vi "Laurel Rate Total TCP.vi"(6 "Laurel Communication Type":string, 8 "error in (no error)":errorcluster, 10 "Measurments in":T7={"Power Measurements"={"Current (A):Element 1"=0.0, "Current (A):Element 2"=0.0, "Power (W):Sigma"=0.0, "Watt Hours (Wh):Sigma"=0.0, "Voltage (V):Element 2"=0.0, "Voltage (V):Element 1"=0.0, "Current Crest Factor:Element 1"=0.0, "Current Crest Factor:Element 2"=0.0, "Voltage Harmonic (%):Element 1"=0.0, "Voltage Harmonic (%):Element 2"=0.0, "Voltage Crest Factor:Element 1"=0.0, "Voltage Crest Factor:Element 2"=0.0, "Time:Element 1"=0.0, "Frequency (Hz):Element 1"=0.0, "Apparent Power (VA):Element 1"=0.0, "Apparent Power (VA):Element 2"=0.0, "Power Factor:Element 1"=0.0, "Power Factor:Element 2"=0.0, "Max Watt Hours"=0.0, "Voltage (V):Element 2 Avg"=0.0, "Voltage (V):Element 1 Avg"=0.0}, "Standby Power"={"Standby Power Spreadsheet"=[], "Standby Power - Pia (Watts)"=0.0, "Off Mode Power - Poff (Watts)"=0.0, "Sia hr/yr"=8620.0, "Soff hr/yr"=0.0, "Yearly Energy Etso kWh/yr"=0.0, "Maximum Power (Watts)"=0.0, "Power Variation (%)"=0.0, "Slope (mW/hr)"=0.0, "Final Harmonics-U1 (%)"="", "Final Harmonics-U2 (%)"="", "Energy (Wh)"=0.0}, "Washer"={"Washer String Data"=[], "Analog Scale Weight (lbs)"=0.0}, "Dishwasher"={"Drain Solonoid Event"=0, "Pump Event"=0, "Water Valve Event"=0, "Heater Event"=0, "Motor Event"=0, "Turbidity Sensor"=0.0, "Spare 2"=0.0, "Spare 3"=0.0, "Spare 4"=0.0, "Spare 5"=0.0, "Thermocouple 1"=0.0, "Thermocouple 2"=0.0, "Thermocouple 3"=0.0, "Thermocouple 4"=0.0, "Thermocouple 5"=0.0, "Thermocouple 6"=0.0, "Spare 1"=0.0, "Dishwasher String Data"=[]}, "Washer HCC"={"Chan 101"=0.0, "Chan 102"=0.0, "Chan 103"=0.0, "Chan 104"=0.0, "Chan 105"=0.0, "Chan 106"=0.0, "Chan 107"=0.0, "Chan 108"=0.0, "Chan 109"=0.0, "Chan 110"=0.0, "Chan 111"=0.0, "Chan 112"=0.0, "Chan 113"=0.0, "Chan 114"=0.0, "Chan 115"=0.0, "Chan 116"=0.0, "Chan 117"=0.0, "Chan 118"=0.0, "Chan 119"=0.0, "Chan 120"=0.0, "Chan 201"=0.0, "Chan 202"=0.0, "Chan 203"=0.0, "Chan 204"=0.0, "Chan 205"=0.0, "Chan 206"=0.0, "Chan 207"=0.0, "Chan 208"=0.0, "Chan 209"=0.0, "Chan 210"=0.0, "Chan 211"=0.0, "Chan 212"=0.0, "Chan 213"=0.0, "Chan 214"=0.0, "Chan 215"=0.0, "Chan 216"=0.0, "Chan 217"=0.0, "Chan 218"=0.0, "Chan 219"=0.0, "Chan 220"=0.0, "Chan 301"=0.0, "Chan 302"=0.0, "Chan 303"=0.0, "Chan 304"=0.0, "Chan 305"=0.0, "Chan 306"=0.0, "Chan 307"=0.0, "Chan 308"=0.0, "Chan 309"=0.0, "Chan 310"=0.0, "Chan 311"=0.0, "Chan 312"=0.0, "Chan 313"=0.0, "Chan 314"=0.0, "Chan 315"=0.0, "Chan 316"=0.0, "Chan 317"=0.0, "Chan 318"=0.0, "Chan 319"=0.0, "Chan 320"=0.0}, "Barometric Pressure"={"Barometric Pressure (in. Hg)"=0.0}, "Ambient Conditions"={"Ambient Temperature  1 (°F)"=0.0, "Ambient Temperature 2 (°F)"=0.0, "Ambient Temperature 3 (°F)"=0.0, "Ambient Humidity 1 (%)"=0.0, "Ambient Humidity 2 (%)"=0.0, "Ambient Humidity 3 (%)"=0.0, "Ambient Dewpoint  1 (°F)"=0.0, "Ambient Dewpoint 2 (°F)"=0.0, "Ambient Dewpoint 3 (°F)"=0.0}, "Weight Scale"={"Gross Weigth (lbs)"=0.0, "Net Weight (lbs)"=0.0, "Final Weight (lbs)"=""}, "Water Measurements"={"Hot Water Pressure (psi)"=0.0, "Hot Water Pressure Max (psi)"=0.0, "Hot Water Temperature (°F)"=0.0, "Cold Water Pressure (psi)"=0.0, "Cold Water Pressure Max (psi)"=0.0, "Hot Water Temperature Max (°F)"=0.0, "Cold Water Temperature (°F)"=0.0, "Cold Water Temperature Max (°F)"=0.0, "Hot Water Total (Gal)"=0.0, "Hot Water Rate (GPM)"=0.0, "Cold Water Total (Gal)"=0.0, "Cold Water Rate (GPM)"=0.0, "Cold Water Total During Wash (Gal)"=0.0, "Hot Water Total During Wash (Gal)"=0.0, "Rinse Cold (Gal)"=0.0, "Rinse Hot (Gal)"=0.0, "Hot Water Pressure Min (psi)"=0.0, "Hot Water Temperature Min (°F)"=0.0, "Cold Water Pressure Min (psi)"=0.0, "Cold Water Temperature Min (°F)"=0.0}, "Gas Data"={"Meter Type (Gas)"="", "Meter ID"=enum."Disabled", "Heating Value (BTU/ft³)"=0.0, "Ft³ / Hr (SCFH)"=0.0, "15 Second Average (BTU/HR)"=0.0, "30 Second Average (BTU/HR)"=0.0, "SLPM (Mass Flow)"=0.0, "LPM (Vol. Flow)"=0.0, "Gas Temperature (°F)"=0.0, "Gas Pressure (PSIA)"=0.0, "Tot.Flow (Liters)"=0.0}} {"Power Measurements"."Voltage (V):Element 1 Avg" format="%.3g"; "Power Measurements"."Voltage (V):Element 2 Avg" format="%.3g"; "Power Measurements"."Max Watt Hours" format="%.3g"; "Power Measurements"."Power Factor:Element 2" format="%.3g"; "Power Measurements"."Power Factor:Element 1" format="%.3g"; "Power Measurements"."Apparent Power (VA):Element 2" format="%.3g"; "Power Measurements"."Apparent Power (VA):Element 1" format="%.3g"; "Power Measurements"."Frequency (Hz):Element 1" format="%.3g"; "Power Measurements"."Time:Element 1" format="%.3g"; "Power Measurements"."Voltage Crest Factor:Element 2" format="%.3g"; "Power Measurements"."Voltage Crest Factor:Element 1" format="%.3g"; "Power Measurements"."Voltage Harmonic (%):Element 2" format="%.3g"; "Power Measurements"."Voltage Harmonic (%):Element 1" format="%.3g"; "Power Measurements"."Current Crest Factor:Element 2" format="%.3g"; "Power Measurements"."Current Crest Factor:Element 1" format="%.3g"; "Power Measurements"."Voltage (V):Element 1" format="%.3g"; "Power Measurements"."Voltage (V):Element 2" format="%.3g"; "Power Measurements"."Watt Hours (Wh):Sigma" format="%.3f"; "Power Measurements"."Power (W):Sigma" format="%.3g"; "Power Measurements"."Current (A):Element 2" format="%.3g"; "Power Measurements"."Current (A):Element 1" format="%.3g"}, 11 "Fixture Hardware in":T1={"Power "={"Yokogawa"={"WT210"={"Sample Rate (1: 0.25s)"=0, "A Range (12: 20A)"=0, "V Range (6: 600V)"=0, "Power VISA Yokogawa WT210"=""}, "WT500"={"Power VISA Yokogawa WT500"="", "V Range (8: 1000V)"=0, "I Range (7: 40A)"=0, "Update Rate (3: 500ms)"=0}, "WT310_2"={"Sample Rate (1: 0.25s)"=1, "A Range (12: 20A)"=11, "V Range (6: 600V)"=4, "Power VISA Yokogawa WT310_2"=""}, "WT310_3"={"Sample Rate (1: 0.25s)"=1, "A Range (12: 20A)"=11, "V Range (6: 600V)"=4, "Power VISA Yokogawa WT310_3"=""}}, "Aplus"={"Aplus IP Address"="", "Remote Port"=0, "Instrument"="", "Instr Driver Revision"=""}, "Power Limits"={"Crest Factor"={"Upper Limit"=0.0, "Lower Limit"=0.0}, "Harmonic Content"={"Uthd"=0.0}, "Voltage"={"% Error"=0.0}, "Stability"={"<1 Watt "={"Wattage"=0.0, "Slope (mW/H)"=0.0}, ">1 Watt"={"1%Power/Hour"=0.0}}}, "Nominal Voltage"=0, "Time Limit (s)"=0.0, "Power Variation Limit (%)"=0.0, "Power Supply"={"Chroma 61605"="", "Use Chroma?"=FALSE}}, "Weight Scale"={"Com Options"={"IND560Scale VISA"="", "IP Address"="", "Remote Port"=0, "Setra Scale VISA"="MW100", "GSE 350"="GSE350"}, "Select Scale"=""}, "Flow Rates"={"Laurel Cold IP Address"="", "Laurel Hot IP Address"="", "Hot Water Laurel VISA"="", "Cold Water Laurel VISA"="", "Remote Port"=0, "Laurel Communication Type"="", "Meters To Collect (Hot Cold)"="", "HOT Laurel Reference"=refnum, "COLD Laurel Reference"=refnum}, "Analog Data"={"Agilent"={"Agilent 34972_1"="", "Agilent 34972_2"="", "Agilent 34972_3"="", "Agilent 34972_4"="", "Agilent 34972_5"="", "Agilent 34972_6"="", "Agilent Gain"=0.0, "TC Type (K,J,T)"="", "Instrument IDN?"="", "TC Channels-List"="", "Analog Channels-List"="", "Agilent Cluster Array"=[], "TC Channels-List 2"="", "Analog Channels-List 2"=""}, "Yokogawa"={"MW100"="", "Intellifaucet"=FALSE}, "Select Analog"="", "TC Coefficients"={"TC Coefficients 1"=[], "TC Coefficients 2"=[], "TC Coefficients 3"=[], "TC Coefficients 4"=[], "TC Coefficients 5"=[], "TC Coefficients 6"=[], "TC Coefficients 7"=[]}, "NI Tasks (Dryer DOE)"=["TC Temps-Module 1", "TC Temps-Module 2", "TC Temps-Module 3", "TC Temps-Module 4", "TC Temps-Module 5", "Gas and Temp-Module 6", "AC_DC Events-Module 7"], "Laurel Analog"={"Laurel IP (Water Temp)"="", "Laurel IP (Pressure)"=""}}, "ITHX-Temp Humidity"={"IP Address 1"="", "Remote Port"=0, "IP Address 2"="", "IP Address 3"=""}, "Gas Meter COM Ports"={"Gas Meter 1"="COM3", "Gas Meter 2"="COM4", "Gas Meter 3"="COM5", "Gas Meter 4"="COM6", "Gas Meter 5"="COM7", "Gas Meter 6"="COM8"}, "Barometric Pressure"={"HEISE 901A"="HEISE", "Use Barometer?"=FALSE}} {"Power"."Yokogawa"."WT310_3"."V Range (6: 600V)" items=["Auto", "15V", "30V", "60V", "150V", "300V", "600V"]; "Power"."Yokogawa"."WT310_3"."A Range (12: 20A)" items=["Auto", "5mA", "10mA", "20mA", "50mA", "100mA", "200mA", "0.5A", "1A", "2A", "5A", "10A", "20A", "50mV", "100mV", "200mV", "2.5V", "5V", "10V"]; "Power"."Yokogawa"."WT310_3"."Sample Rate (1: 0.25s)" items=["0.1s", "0.25s", "0.5s", "1s", "2s", "5s"]; "Power"."Yokogawa"."WT310_2"."V Range (6: 600V)" items=["Auto", "15V", "30V", "60V", "150V", "300V", "600V"]; "Power"."Yokogawa"."WT310_2"."A Range (12: 20A)" items=["Auto", "5mA", "10mA", "20mA", "50mA", "100mA", "200mA", "0.5A", "1A", "2A", "5A", "10A", "20A", "50mV", "100mV", "200mV", "2.5V", "5V", "10V"]; "Power"."Yokogawa"."WT310_2"."Sample Rate (1: 0.25s)" items=["0.1s", "0.25s", "0.5s", "1s", "2s", "5s"]; "Power"."Yokogawa"."WT500"."Update Rate (3: 500ms)" items=["-", "100ms", "200ms", "500ms", "1s", "2s", "5s"]; "Power"."Yokogawa"."WT500"."I Range (7: 40A)" items=["AUTO", "500 mA", "1 A", "2 A", "5 A", "10 A", "20 A", "40 A", "S-AUTO", "50 mV", "100 mV", "200 mV", "500 mV", "1 V", "2 V", "5 V", "10 V", "250 mA", "500 mA", "1 A", "2.5 A", "5 A", "10 A", "20 A", "25 mV", "50 mV", "100 mV", "250 mV", "500 mV", "1 V", "2.5 V", "5 V"]; "Power"."Yokogawa"."WT500"."V Range (8: 1000V)" items=["AUTO", "15", "30", "60", "100", "150", "300", "600", "1000", "7.5", "15", "30", "50", "75", "150", "300", "500"]; "Power"."Yokogawa"."WT210"."V Range (6: 600V)" items=["Auto", "15V", "30V", "60V", "150V", "300V", "600V"]; "Power"."Yokogawa"."WT210"."A Range (12: 20A)" items=["Auto", "5mA", "10mA", "20mA", "50mA", "100mA", "200mA", "0.5A", "1A", "2A", "5A", "10A", "20A", "50mV", "100mV", "200mV", "2.5V", "5V", "10V"]; "Power"."Yokogawa"."WT210"."Sample Rate (1: 0.25s)" items=["0.1s", "0.25s", "0.5s", "1s", "2s", "5s"]}) -> (0 "error out":errorcluster, 2 "Measurments out":T7={"Power Measurements"={"Current (A):Element 1"=0.0, "Current (A):Element 2"=0.0, "Power (W):Sigma"=0.0, "Watt Hours (Wh):Sigma"=0.0, "Voltage (V):Element 2"=0.0, "Voltage (V):Element 1"=0.0, "Current Crest Factor:Element 1"=0.0, "Current Crest Factor:Element 2"=0.0, "Voltage Harmonic (%):Element 1"=0.0, "Voltage Harmonic (%):Element 2"=0.0, "Voltage Crest Factor:Element 1"=0.0, "Voltage Crest Factor:Element 2"=0.0, "Time:Element 1"=0.0, "Frequency (Hz):Element 1"=0.0, "Apparent Power (VA):Element 1"=0.0, "Apparent Power (VA):Element 2"=0.0, "Power Factor:Element 1"=0.0, "Power Factor:Element 2"=0.0, "Max Watt Hours"=0.0, "Voltage (V):Element 2 Avg"=0.0, "Voltage (V):Element 1 Avg"=0.0}, "Standby Power"={"Standby Power Spreadsheet"=[], "Standby Power - Pia (Watts)"=0.0, "Off Mode Power - Poff (Watts)"=0.0, "Sia hr/yr"=8620.0, "Soff hr/yr"=0.0, "Yearly Energy Etso kWh/yr"=0.0, "Maximum Power (Watts)"=0.0, "Power Variation (%)"=0.0, "Slope (mW/hr)"=0.0, "Final Harmonics-U1 (%)"="", "Final Harmonics-U2 (%)"="", "Energy (Wh)"=0.0}, "Washer"={"Washer String Data"=[], "Analog Scale Weight (lbs)"=0.0}, "Dishwasher"={"Drain Solonoid Event"=0, "Pump Event"=0, "Water Valve Event"=0, "Heater Event"=0, "Motor Event"=0, "Turbidity Sensor"=0.0, "Spare 2"=0.0, "Spare 3"=0.0, "Spare 4"=0.0, "Spare 5"=0.0, "Thermocouple 1"=0.0, "Thermocouple 2"=0.0, "Thermocouple 3"=0.0, "Thermocouple 4"=0.0, "Thermocouple 5"=0.0, "Thermocouple 6"=0.0, "Spare 1"=0.0, "Dishwasher String Data"=[]}, "Washer HCC"={"Chan 101"=0.0, "Chan 102"=0.0, "Chan 103"=0.0, "Chan 104"=0.0, "Chan 105"=0.0, "Chan 106"=0.0, "Chan 107"=0.0, "Chan 108"=0.0, "Chan 109"=0.0, "Chan 110"=0.0, "Chan 111"=0.0, "Chan 112"=0.0, "Chan 113"=0.0, "Chan 114"=0.0, "Chan 115"=0.0, "Chan 116"=0.0, "Chan 117"=0.0, "Chan 118"=0.0, "Chan 119"=0.0, "Chan 120"=0.0, "Chan 201"=0.0, "Chan 202"=0.0, "Chan 203"=0.0, "Chan 204"=0.0, "Chan 205"=0.0, "Chan 206"=0.0, "Chan 207"=0.0, "Chan 208"=0.0, "Chan 209"=0.0, "Chan 210"=0.0, "Chan 211"=0.0, "Chan 212"=0.0, "Chan 213"=0.0, "Chan 214"=0.0, "Chan 215"=0.0, "Chan 216"=0.0, "Chan 217"=0.0, "Chan 218"=0.0, "Chan 219"=0.0, "Chan 220"=0.0, "Chan 301"=0.0, "Chan 302"=0.0, "Chan 303"=0.0, "Chan 304"=0.0, "Chan 305"=0.0, "Chan 306"=0.0, "Chan 307"=0.0, "Chan 308"=0.0, "Chan 309"=0.0, "Chan 310"=0.0, "Chan 311"=0.0, "Chan 312"=0.0, "Chan 313"=0.0, "Chan 314"=0.0, "Chan 315"=0.0, "Chan 316"=0.0, "Chan 317"=0.0, "Chan 318"=0.0, "Chan 319"=0.0, "Chan 320"=0.0}, "Barometric Pressure"={"Barometric Pressure (in. Hg)"=0.0}, "Ambient Conditions"={"Ambient Temperature  1 (°F)"=0.0, "Ambient Temperature 2 (°F)"=0.0, "Ambient Temperature 3 (°F)"=0.0, "Ambient Humidity 1 (%)"=0.0, "Ambient Humidity 2 (%)"=0.0, "Ambient Humidity 3 (%)"=0.0, "Ambient Dewpoint  1 (°F)"=0.0, "Ambient Dewpoint 2 (°F)"=0.0, "Ambient Dewpoint 3 (°F)"=0.0}, "Weight Scale"={"Gross Weigth (lbs)"=0.0, "Net Weight (lbs)"=0.0, "Final Weight (lbs)"=""}, "Water Measurements"={"Hot Water Pressure (psi)"=0.0, "Hot Water Pressure Max (psi)"=0.0, "Hot Water Temperature (°F)"=0.0, "Cold Water Pressure (psi)"=0.0, "Cold Water Pressure Max (psi)"=0.0, "Hot Water Temperature Max (°F)"=0.0, "Cold Water Temperature (°F)"=0.0, "Cold Water Temperature Max (°F)"=0.0, "Hot Water Total (Gal)"=0.0, "Hot Water Rate (GPM)"=0.0, "Cold Water Total (Gal)"=0.0, "Cold Water Rate (GPM)"=0.0, "Cold Water Total During Wash (Gal)"=0.0, "Hot Water Total During Wash (Gal)"=0.0, "Rinse Cold (Gal)"=0.0, "Rinse Hot (Gal)"=0.0, "Hot Water Pressure Min (psi)"=0.0, "Hot Water Temperature Min (°F)"=0.0, "Cold Water Pressure Min (psi)"=0.0, "Cold Water Temperature Min (°F)"=0.0}, "Gas Data"={"Meter Type (Gas)"="", "Meter ID"=enum."Disabled", "Heating Value (BTU/ft³)"=0.0, "Ft³ / Hr (SCFH)"=0.0, "15 Second Average (BTU/HR)"=0.0, "30 Second Average (BTU/HR)"=0.0, "SLPM (Mass Flow)"=0.0, "LPM (Vol. Flow)"=0.0, "Gas Temperature (°F)"=0.0, "Gas Pressure (PSIA)"=0.0, "Tot.Flow (Liters)"=0.0}} {"Power Measurements"."Voltage (V):Element 1 Avg" format="%.3g"; "Power Measurements"."Voltage (V):Element 2 Avg" format="%.3g"; "Power Measurements"."Max Watt Hours" format="%.3g"; "Power Measurements"."Power Factor:Element 2" format="%.3g"; "Power Measurements"."Power Factor:Element 1" format="%.3g"; "Power Measurements"."Apparent Power (VA):Element 2" format="%.3g"; "Power Measurements"."Apparent Power (VA):Element 1" format="%.3g"; "Power Measurements"."Frequency (Hz):Element 1" format="%.3g"; "Power Measurements"."Time:Element 1" format="%.3g"; "Power Measurements"."Voltage Crest Factor:Element 2" format="%.3g"; "Power Measurements"."Voltage Crest Factor:Element 1" format="%.3g"; "Power Measurements"."Voltage Harmonic (%):Element 2" format="%.3g"; "Power Measurements"."Voltage Harmonic (%):Element 1" format="%.3g"; "Power Measurements"."Current Crest Factor:Element 2" format="%.3g"; "Power Measurements"."Current Crest Factor:Element 1" format="%.3g"; "Power Measurements"."Voltage (V):Element 1" format="%.3g"; "Power Measurements"."Voltage (V):Element 2" format="%.3g"; "Power Measurements"."Watt Hours (Wh):Sigma" format="%.3f"; "Power Measurements"."Power (W):Sigma" format="%.3g"; "Power Measurements"."Current (A):Element 2" format="%.3g"; "Power Measurements"."Current (A):Element 1" format="%.3g"}, 3 "Fixture Hardware out":T1={"Power "={"Yokogawa"={"WT210"={"Sample Rate (1: 0.25s)"=0, "A Range (12: 20A)"=0, "V Range (6: 600V)"=0, "Power VISA Yokogawa WT210"=""}, "WT500"={"Power VISA Yokogawa WT500"="", "V Range (8: 1000V)"=0, "I Range (7: 40A)"=0, "Update Rate (3: 500ms)"=0}, "WT310_2"={"Sample Rate (1: 0.25s)"=1, "A Range (12: 20A)"=11, "V Range (6: 600V)"=4, "Power VISA Yokogawa WT310_2"=""}, "WT310_3"={"Sample Rate (1: 0.25s)"=1, "A Range (12: 20A)"=11, "V Range (6: 600V)"=4, "Power VISA Yokogawa WT310_3"=""}}, "Aplus"={"Aplus IP Address"="", "Remote Port"=0, "Instrument"="", "Instr Driver Revision"=""}, "Power Limits"={"Crest Factor"={"Upper Limit"=0.0, "Lower Limit"=0.0}, "Harmonic Content"={"Uthd"=0.0}, "Voltage"={"% Error"=0.0}, "Stability"={"<1 Watt "={"Wattage"=0.0, "Slope (mW/H)"=0.0}, ">1 Watt"={"1%Power/Hour"=0.0}}}, "Nominal Voltage"=0, "Time Limit (s)"=0.0, "Power Variation Limit (%)"=0.0, "Power Supply"={"Chroma 61605"="", "Use Chroma?"=FALSE}}, "Weight Scale"={"Com Options"={"IND560Scale VISA"="", "IP Address"="", "Remote Port"=0, "Setra Scale VISA"="MW100", "GSE 350"="GSE350"}, "Select Scale"=""}, "Flow Rates"={"Laurel Cold IP Address"="", "Laurel Hot IP Address"="", "Hot Water Laurel VISA"="", "Cold Water Laurel VISA"="", "Remote Port"=0, "Laurel Communication Type"="", "Meters To Collect (Hot Cold)"="", "HOT Laurel Reference"=refnum, "COLD Laurel Reference"=refnum}, "Analog Data"={"Agilent"={"Agilent 34972_1"="", "Agilent 34972_2"="", "Agilent 34972_3"="", "Agilent 34972_4"="", "Agilent 34972_5"="", "Agilent 34972_6"="", "Agilent Gain"=0.0, "TC Type (K,J,T)"="", "Instrument IDN?"="", "TC Channels-List"="", "Analog Channels-List"="", "Agilent Cluster Array"=[], "TC Channels-List 2"="", "Analog Channels-List 2"=""}, "Yokogawa"={"MW100"="", "Intellifaucet"=FALSE}, "Select Analog"="", "TC Coefficients"={"TC Coefficients 1"=[], "TC Coefficients 2"=[], "TC Coefficients 3"=[], "TC Coefficients 4"=[], "TC Coefficients 5"=[], "TC Coefficients 6"=[], "TC Coefficients 7"=[]}, "NI Tasks (Dryer DOE)"=["TC Temps-Module 1", "TC Temps-Module 2", "TC Temps-Module 3", "TC Temps-Module 4", "TC Temps-Module 5", "Gas and Temp-Module 6", "AC_DC Events-Module 7"], "Laurel Analog"={"Laurel IP (Water Temp)"="", "Laurel IP (Pressure)"=""}}, "ITHX-Temp Humidity"={"IP Address 1"="", "Remote Port"=0, "IP Address 2"="", "IP Address 3"=""}, "Gas Meter COM Ports"={"Gas Meter 1"="COM3", "Gas Meter 2"="COM4", "Gas Meter 3"="COM5", "Gas Meter 4"="COM6", "Gas Meter 5"="COM7", "Gas Meter 6"="COM8"}, "Barometric Pressure"={"HEISE 901A"="HEISE", "Use Barometer?"=FALSE}} {"Power"."Yokogawa"."WT310_3"."V Range (6: 600V)" items=["Auto", "15V", "30V", "60V", "150V", "300V", "600V"]; "Power"."Yokogawa"."WT310_3"."A Range (12: 20A)" items=["Auto", "5mA", "10mA", "20mA", "50mA", "100mA", "200mA", "0.5A", "1A", "2A", "5A", "10A", "20A", "50mV", "100mV", "200mV", "2.5V", "5V", "10V"]; "Power"."Yokogawa"."WT310_3"."Sample Rate (1: 0.25s)" items=["0.1s", "0.25s", "0.5s", "1s", "2s", "5s"]; "Power"."Yokogawa"."WT310_2"."V Range (6: 600V)" items=["Auto", "15V", "30V", "60V", "150V", "300V", "600V"]; "Power"."Yokogawa"."WT310_2"."A Range (12: 20A)" items=["Auto", "5mA", "10mA", "20mA", "50mA", "100mA", "200mA", "0.5A", "1A", "2A", "5A", "10A", "20A", "50mV", "100mV", "200mV", "2.5V", "5V", "10V"]; "Power"."Yokogawa"."WT310_2"."Sample Rate (1: 0.25s)" items=["0.1s", "0.25s", "0.5s", "1s", "2s", "5s"]; "Power"."Yokogawa"."WT500"."Update Rate (3: 500ms)" items=["-", "100ms", "200ms", "500ms", "1s", "2s", "5s"]; "Power"."Yokogawa"."WT500"."I Range (7: 40A)" items=["AUTO", "500 mA", "1 A", "2 A", "5 A", "10 A", "20 A", "40 A", "S-AUTO", "50 mV", "100 mV", "200 mV", "500 mV", "1 V", "2 V", "5 V", "10 V", "250 mA", "500 mA", "1 A", "2.5 A", "5 A", "10 A", "20 A", "25 mV", "50 mV", "100 mV", "250 mV", "500 mV", "1 V", "2.5 V", "5 V"]; "Power"."Yokogawa"."WT500"."V Range (8: 1000V)" items=["AUTO", "15", "30", "60", "100", "150", "300", "600", "1000", "7.5", "15", "30", "50", "75", "150", "300", "500"]; "Power"."Yokogawa"."WT210"."V Range (6: 600V)" items=["Auto", "15V", "30V", "60V", "150V", "300V", "600V"]; "Power"."Yokogawa"."WT210"."A Range (12: 20A)" items=["Auto", "5mA", "10mA", "20mA", "50mA", "100mA", "200mA", "0.5A", "1A", "2A", "5A", "10A", "20A", "50mV", "100mV", "200mV", "2.5V", "5V", "10V"]; "Power"."Yokogawa"."WT210"."Sample Rate (1: 0.25s)" items=["0.1s", "0.25s", "0.5s", "1s", "2s", "5s"]})   [LabVIEW 2018]
uses:
  Trunk/Washer DOE/Type Definitions/DOE Front Panel Meters.ctl
  Trunk/Utility/Type Definitions/UTILITY Power Data.ctl
  Trunk/Utility/Standby Power/Type Definitions/Standby Power Main Data.ctl
  Omega FMA-1600A Series Gas Flow Meter/Type Definitions/FMA1600A Gas Data.ctl
  Omega FMA-1600A Series Gas Flow Meter/Type Definitions/FMA1600A Gas Type.ctl
  Trunk/Range/Type Definitions/RANGE Meter Selector 1-2.ctl
  Trunk/Washer DOE/Type Definitions/DOE Test Fixture Hardware.ctl
  Trunk/Utility/Type Definitions/UTILITY Power Inputs Control.ctl
  IND560 Scale Monitor/Type Definitions/IND560 Configuration.ctl
  Trunk/Hybrid Water Heater/Type Definitions/HEWH Agilent Cluster.ctl
  Trunk/Utility/Type Definitions/UTILITY TC Coefficients.ctl
  Omega FMA-1600A Series Gas Flow Meter/Type Definitions/FMA1600A COM Ports.ctl
  Type Definitions/Laurel Serial Commands.ctl
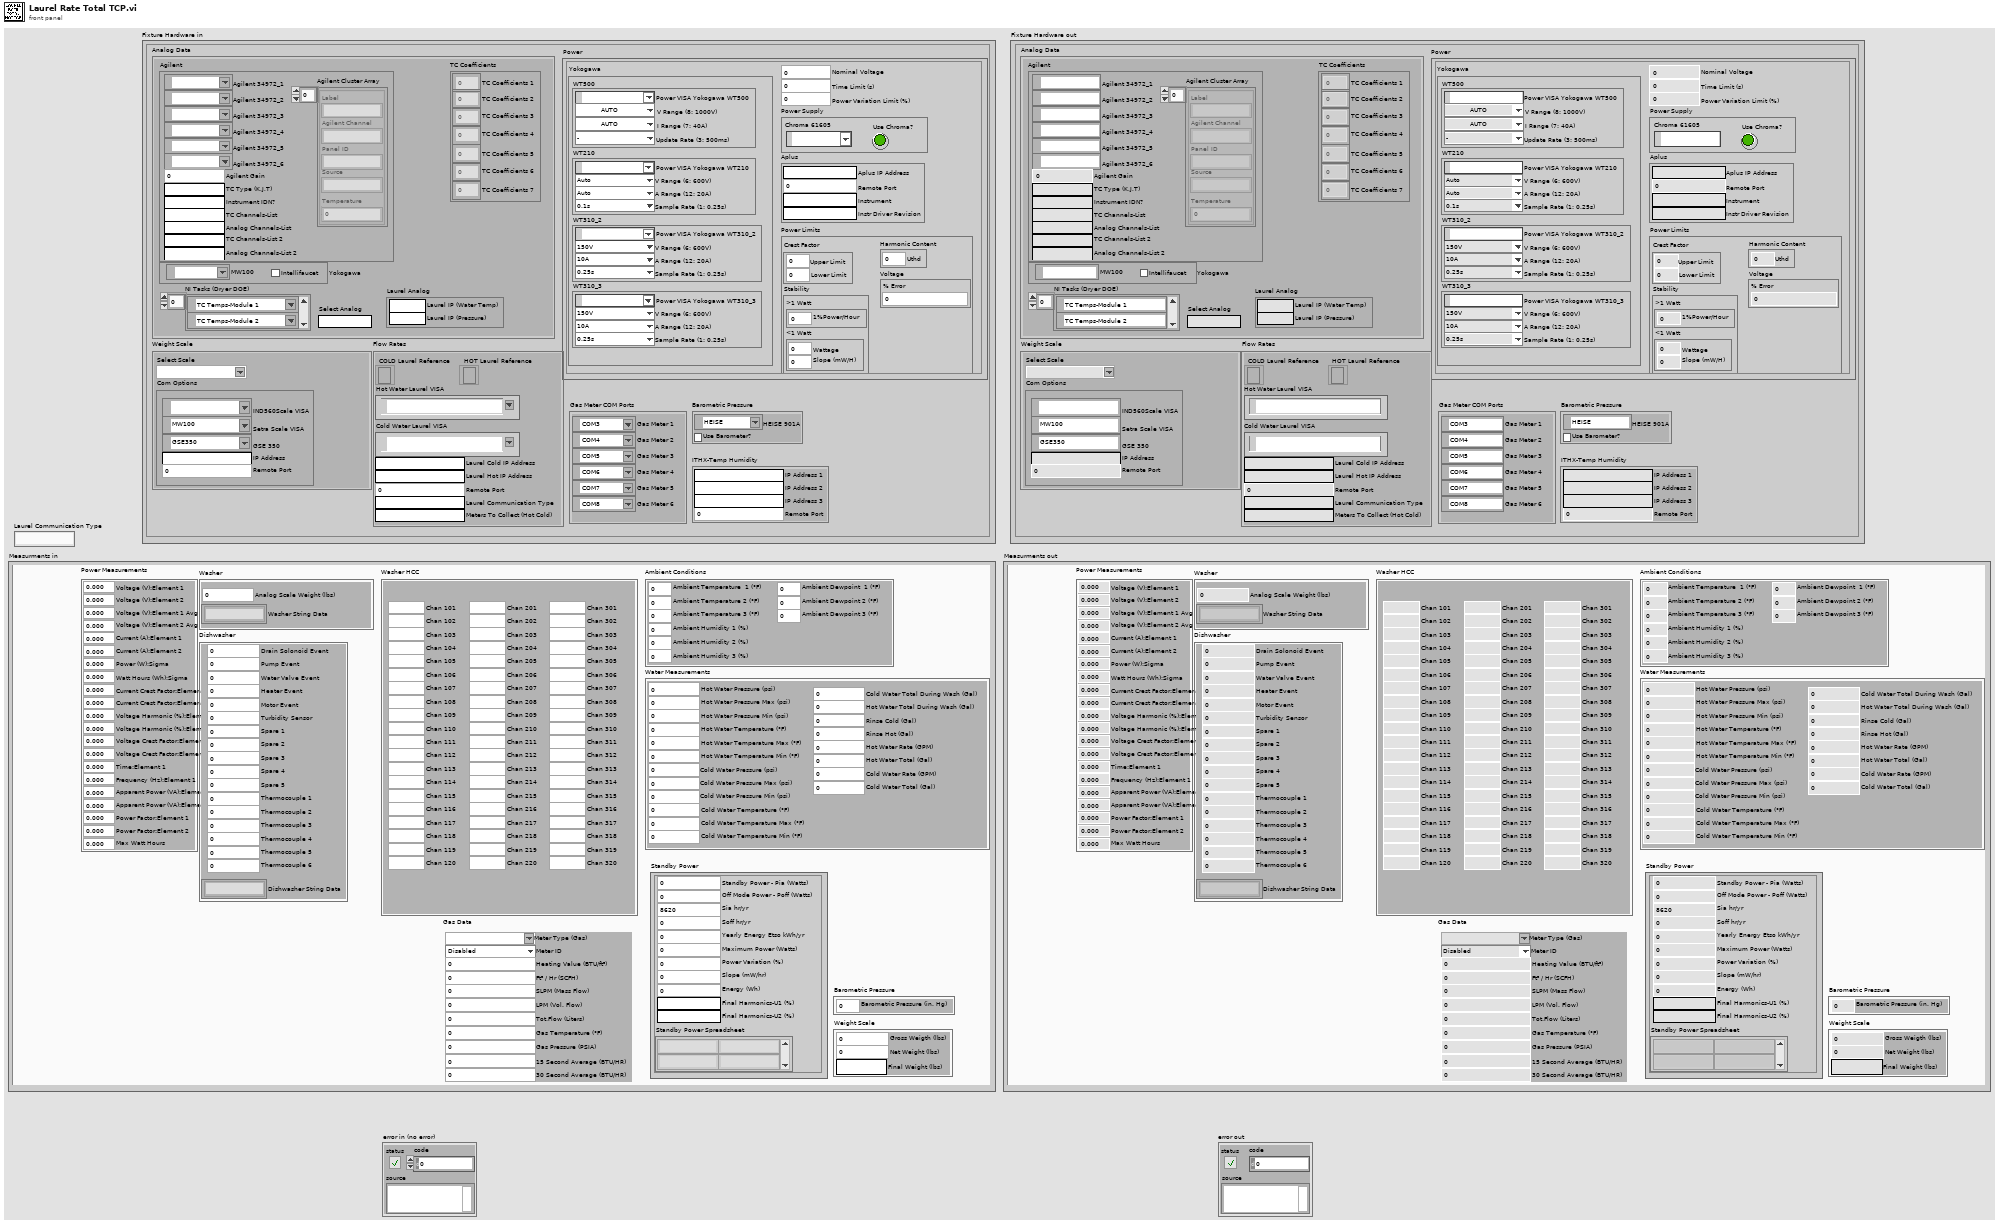
[diagram p1: front panel]
types:
  T1 = typedef "DOE Test Fixture Hardware.ctl" = cluster{"Power ":T2, "Weight Scale":cluster{"Com Options":T3, "Select Scale":string}, "Flow Rates":cluster{"Laurel Cold IP Address":string, "Laurel Hot IP Address":string, "Hot Water Laurel VISA":refnum<visa-resource-name>, "Cold Water Laurel VISA":refnum<visa-resource-name>, "Remote Port":u16, "Laurel Communication Type":string, "Meters To Collect (Hot Cold)":string, "HOT Laurel Reference":refnum<k5>, "COLD Laurel Reference":refnum<k5>}, "Analog Data":cluster{"Agilent":cluster{"Agilent 34972_1":refnum<visa-resource-name>, "Agilent 34972_2":refnum<visa-resource-name>, "Agilent 34972_3":refnum<visa-resource-name>, "Agilent 34972_4":refnum<visa-resource-name>, "Agilent 34972_5":refnum<visa-resource-name>, "Agilent 34972_6":refnum<visa-resource-name>, "Agilent Gain":dbl, "TC Type (K,J,T)":string, "Instrument IDN?":string, "TC Channels-List":string, "Analog Channels-List":string, "Agilent Cluster Array":T4[], "TC Channels-List 2":string, "Analog Channels-List 2":string}, "Yokogawa":cluster{"MW100":refnum<visa-resource-name>, "Intellifaucet":bool}, "Select Analog":string, "TC Coefficients":T5, "NI Tasks (Dryer DOE)":refnum<k21>[], "Laurel Analog":cluster{"Laurel IP (Water Temp)":string, "Laurel IP (Pressure)":string}}, "ITHX-Temp Humidity":cluster{"IP Address 1":string, "Remote Port":u16, "IP Address 2":string, "IP Address 3":string}, "Gas Meter COM Ports":T6, "Barometric Pressure":cluster{"HEISE 901A":refnum<visa-resource-name>, "Use Barometer?":bool}}
  T2 = typedef "UTILITY Power Inputs Control.ctl" = cluster{"Yokogawa":cluster{"WT210":cluster{"Sample Rate (1: 0.25s)":i32, "A Range (12: 20A)":i32, "V Range (6: 600V)":i32, "Power VISA Yokogawa WT210":refnum<visa-resource-name>}, "WT500":cluster{"Power VISA Yokogawa WT500":refnum<visa-resource-name>, "V Range (8: 1000V)":i32, "I Range (7: 40A)":i32, "Update Rate (3: 500ms)":i32}, "WT310_2":cluster{"Sample Rate (1: 0.25s)":i32, "A Range (12: 20A)":i32, "V Range (6: 600V)":i32, "Power VISA Yokogawa WT310_2":refnum<visa-resource-name>}, "WT310_3":cluster{"Sample Rate (1: 0.25s)":i32, "A Range (12: 20A)":i32, "V Range (6: 600V)":i32, "Power VISA Yokogawa WT310_3":refnum<visa-resource-name>}}, "Aplus":cluster{"Aplus IP Address":string, "Remote Port":i32, "Instrument":string, "Instr Driver Revision":string}, "Power Limits":cluster{"Crest Factor":cluster{"Upper Limit":dbl, "Lower Limit":dbl}, "Harmonic Content":cluster{"Uthd":dbl}, "Voltage":cluster{"% Error":dbl}, "Stability":cluster{"<1 Watt ":cluster{"Wattage":dbl, "Slope (mW/H)":dbl}, ">1 Watt":cluster{"1%Power/Hour":dbl}}}, "Nominal Voltage":i32, "Time Limit (s)":dbl, "Power Variation Limit (%)":dbl, "Power Supply":cluster{"Chroma 61605":refnum<visa-resource-name>, "Use Chroma?":bool}}
  T3 = typedef "IND560 Configuration.ctl" = cluster{"IND560Scale VISA":refnum<visa-resource-name>, "IP Address":string, "Remote Port":u16, "Setra Scale VISA":refnum<visa-resource-name>, "GSE 350":refnum<visa-resource-name>}
  T4 = typedef "HEWH Agilent Cluster.ctl" = cluster{"Label":string, "Agilent Channel":string, "Panel ID":string, "Source":string, "Temperature":dbl}
  T5 = typedef "UTILITY TC Coefficients.ctl" = cluster{"TC Coefficients 1":dbl[], "TC Coefficients 2":dbl[], "TC Coefficients 3":dbl[], "TC Coefficients 4":dbl[], "TC Coefficients 5":dbl[], "TC Coefficients 6":dbl[], "TC Coefficients 7":dbl[]}
  T6 = typedef "FMA1600A COM Ports.ctl" = cluster{"Gas Meter 1":refnum<visa-resource-name>, "Gas Meter 2":refnum<visa-resource-name>, "Gas Meter 3":refnum<visa-resource-name>, "Gas Meter 4":refnum<visa-resource-name>, "Gas Meter 5":refnum<visa-resource-name>, "Gas Meter 6":refnum<visa-resource-name>}
  T7 = typedef "DOE Front Panel Meters.ctl" = cluster{"Power Measurements":T8, "Standby Power":T9, "Washer":cluster{"Washer String Data":string[][], "Analog Scale Weight (lbs)":dbl}, "Dishwasher":cluster{"Drain Solonoid Event":i32, "Pump Event":i32, "Water Valve Event":i32, "Heater Event":i32, "Motor Event":i32, "Turbidity Sensor":dbl, "Spare 2":dbl, "Spare 3":dbl, "Spare 4":dbl, "Spare 5":dbl, "Thermocouple 1":dbl, "Thermocouple 2":dbl, "Thermocouple 3":dbl, "Thermocouple 4":dbl, "Thermocouple 5":dbl, "Thermocouple 6":dbl, "Spare 1":dbl, "Dishwasher String Data":string[][]}, "Washer HCC":cluster{"Chan 101":dbl, "Chan 102":dbl, "Chan 103":dbl, "Chan 104":dbl, "Chan 105":dbl, "Chan 106":dbl, "Chan 107":dbl, "Chan 108":dbl, "Chan 109":dbl, "Chan 110":dbl, "Chan 111":dbl, "Chan 112":dbl, "Chan 113":dbl, "Chan 114":dbl, "Chan 115":dbl, "Chan 116":dbl, "Chan 117":dbl, "Chan 118":dbl, "Chan 119":dbl, "Chan 120":dbl, "Chan 201":dbl, "Chan 202":dbl, "Chan 203":dbl, "Chan 204":dbl, "Chan 205":dbl, "Chan 206":dbl, "Chan 207":dbl, "Chan 208":dbl, "Chan 209":dbl, "Chan 210":dbl, "Chan 211":dbl, "Chan 212":dbl, "Chan 213":dbl, "Chan 214":dbl, "Chan 215":dbl, "Chan 216":dbl, "Chan 217":dbl, "Chan 218":dbl, "Chan 219":dbl, "Chan 220":dbl, "Chan 301":dbl, "Chan 302":dbl, "Chan 303":dbl, "Chan 304":dbl, "Chan 305":dbl, "Chan 306":dbl, "Chan 307":dbl, "Chan 308":dbl, "Chan 309":dbl, "Chan 310":dbl, "Chan 311":dbl, "Chan 312":dbl, "Chan 313":dbl, "Chan 314":dbl, "Chan 315":dbl, "Chan 316":dbl, "Chan 317":dbl, "Chan 318":dbl, "Chan 319":dbl, "Chan 320":dbl}, "Barometric Pressure":cluster{"Barometric Pressure (in. Hg)":dbl}, "Ambient Conditions":cluster{"Ambient Temperature  1 (°F)":dbl, "Ambient Temperature 2 (°F)":dbl, "Ambient Temperature 3 (°F)":dbl, "Ambient Humidity 1 (%)":dbl, "Ambient Humidity 2 (%)":dbl, "Ambient Humidity 3 (%)":dbl, "Ambient Dewpoint  1 (°F)":dbl, "Ambient Dewpoint 2 (°F)":dbl, "Ambient Dewpoint 3 (°F)":dbl}, "Weight Scale":cluster{"Gross Weigth (lbs)":dbl, "Net Weight (lbs)":dbl, "Final Weight (lbs)":string}, "Water Measurements":cluster{"Hot Water Pressure (psi)":dbl, "Hot Water Pressure Max (psi)":dbl, "Hot Water Temperature (°F)":dbl, "Cold Water Pressure (psi)":dbl, "Cold Water Pressure Max (psi)":dbl, "Hot Water Temperature Max (°F)":dbl, "Cold Water Temperature (°F)":dbl, "Cold Water Temperature Max (°F)":dbl, "Hot Water Total (Gal)":dbl, "Hot Water Rate (GPM)":dbl, "Cold Water Total (Gal)":dbl, "Cold Water Rate (GPM)":dbl, "Cold Water Total During Wash (Gal)":dbl, "Hot Water Total During Wash (Gal)":dbl, "Rinse Cold (Gal)":dbl, "Rinse Hot (Gal)":dbl, "Hot Water Pressure Min (psi)":dbl, "Hot Water Temperature Min (°F)":dbl, "Cold Water Pressure Min (psi)":dbl, "Cold Water Temperature Min (°F)":dbl}, "Gas Data":T10}
  T8 = typedef "UTILITY Power Data.ctl" = cluster{"Current (A):Element 1":dbl, "Current (A):Element 2":dbl, "Power (W):Sigma":dbl, "Watt Hours (Wh):Sigma":dbl, "Voltage (V):Element 2":dbl, "Voltage (V):Element 1":dbl, "Current Crest Factor:Element 1":dbl, "Current Crest Factor:Element 2":dbl, "Voltage Harmonic (%):Element 1":dbl, "Voltage Harmonic (%):Element 2":dbl, "Voltage Crest Factor:Element 1":dbl, "Voltage Crest Factor:Element 2":dbl, "Time:Element 1":dbl, "Frequency (Hz):Element 1":dbl, "Apparent Power (VA):Element 1":dbl, "Apparent Power (VA):Element 2":dbl, "Power Factor:Element 1":dbl, "Power Factor:Element 2":dbl, "Max Watt Hours":dbl, "Voltage (V):Element 2 Avg":dbl, "Voltage (V):Element 1 Avg":dbl}
  T9 = typedef "Standby Power Main Data.ctl" = cluster{"Standby Power Spreadsheet":string[][], "Standby Power - Pia (Watts)":dbl, "Off Mode Power - Poff (Watts)":dbl, "Sia hr/yr":dbl, "Soff hr/yr":dbl, "Yearly Energy Etso kWh/yr":dbl, "Maximum Power (Watts)":dbl, "Power Variation (%)":dbl, "Slope (mW/hr)":dbl, "Final Harmonics-U1 (%)":string, "Final Harmonics-U2 (%)":string, "Energy (Wh)":dbl}
  T10 = typedef "FMA1600A Gas Data.ctl" = cluster{"Meter Type (Gas)":T11, "Meter ID":T12, "Heating Value (BTU/ft³)":dbl, "Ft³ / Hr (SCFH)":dbl, "15 Second Average (BTU/HR)":dbl, "30 Second Average (BTU/HR)":dbl, "SLPM (Mass Flow)":dbl, "LPM (Vol. Flow)":dbl, "Gas Temperature (°F)":dbl, "Gas Pressure (PSIA)":dbl, "Tot.Flow (Liters)":dbl}
  T11 = typedef "FMA1600A Gas Type.ctl" = string
  T12 = typedef "RANGE Meter Selector 1-2.ctl" = enum16{"Disabled", "Meter 1", "Meter 2", "Auto"}
  T13 = typedef "Laurel Serial Commands.ctl" = string
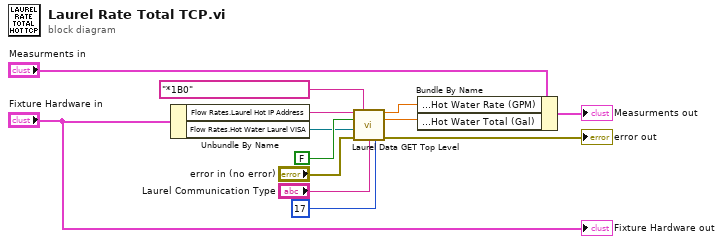
[diagram p0: block diagram]
diagram:
  n1 = Unbundle By Name("Fixture Hardware in") -> ("Flow Rates.Laurel Hot IP Address"=w9:string, "Flow Rates.Hot Water Laurel VISA"=w2:refnum<visa-resource-name>)
  n2 = call "Laurel Data GET Top Level.vi"("Laurel IP Address"=w9, "Laurel Serial Commands"=T13 "*1B0", "Use Delay"=FALSE, "Serial VISA"=w2, "error in (no error)"="error in (no error)", "Laurel Communication Type"="Laurel Communication Type", "All Items Byte Count (Flow Rate)"=17 ("byte count")) -> ("Flow Rate (Item 1)"=w11:dbl, "Gallons (Item 2)"=w10:dbl, "error out"=→"error out":errorcluster)  [unwired: 3 in, 3 out]
  n3 = Bundle By Name(cluster="Measurments in", "Water Measurements.Hot Water Rate (GPM)"=w11, "Water Measurements.Hot Water Total (Gal)"=w10) -> (→"Measurments out":T7)
  "Fixture Hardware out" <- "Fixture Hardware in"
